vi "Anritsu1c_MT8852B_YYLL_Test.vi"(11 "YTESTER测试数据":T1={"Socket(From1)"=1, "SN"=refnum, "StopFlagRef"=refnum, "YT System Queue"=refnum}) -> (3 "YTESTER结论":T2)   [LabVIEW 2017]
doc: "VIDescription=线损设置"
uses:
  YtCommon.lvlibp/yt`Step StepBaseInput.ctl
  YtCommon.lvlibp/yt`Step StepResult.ctl
  YtCommon.lvlibp/yt`Step TestData.ctl
  YtCommon.lvlibp/yt`Step System Queue.ctl
  Step`s VIs/YYLLGeneric/variable_W.ctl
  YtCommon.lvlibp/yt`Data-Ytester Type Data.ctl
  Step`s VIs/YYLLIdea/yyllMT8852B/Anritsu_MT8852B_YYLL_Result.ctl
  <vilib>/regexp/Match Regular Expression.xnode
  YtCommon.lvlibp
panel:
  in  "YTESTER开放参数":T4={"YTESTER_BaseInput"={"isTest"=TRUE, "isSkip"=FALSE, "StepName"="AnritsuMT8852B测试", "OnPass"=enum."Next", "OnFail"=enum."Next", "ReTestNumber"=0.0}, "VISA resource name"="", "测试MAC来源"=enum."搜索测试", "指定MAC"="", "Test Timeout(s)"=30.0}
  # "#yyll 建议\n蓝牙测试繁多！测试Maybe只对生产工艺过程导致异常排筛、效率负责，无需过多专业测试。"
  # "MT8852B"
  # "Anritsu"
  # "YYLL"
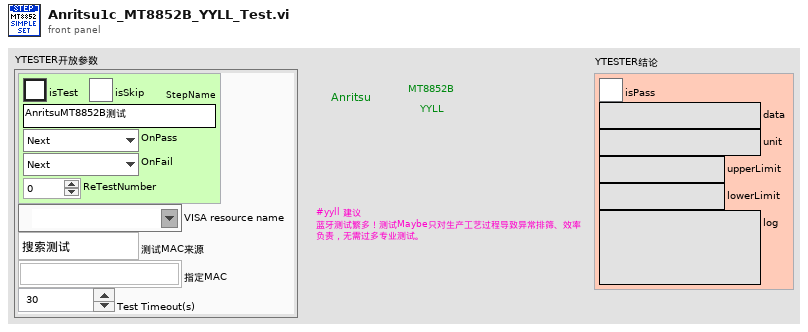
[diagram p1: front panel]
types:
  T1 = typedef "YtCommon.lvlibp/yt`Step TestData.ctl" = cluster{"Socket(From1)":i32, "SN":refnum<notifier>, "StopFlagRef":refnum<notifier>, "YT System Queue":refnum<queue>}
  T2 = typedef "YtCommon.lvlibp/yt`Step StepResult.ctl" = cluster{"isPass":bool, "data":string, "unit":string, "upperLimit":string, "lowerLimit":string, "log":string}
  T3 = typedef "YtCommon.lvlibp/yt`Step StepBaseInput.ctl" = cluster{"isTest":bool, "isSkip":bool, "StepName":string, "OnPass":enum16{"Next", "ToOVER", "Terminate"}, "OnFail":enum16{"Next", "ToOVER", "Terminate"}, "ReTestNumber":dbl}
  T4 = cluster{"YTESTER_BaseInput":T3, "VISA resource name":refnum<visa-resource-name>, "测试MAC来源":enum16{"搜索测试", "指定MAC测试"}, "指定MAC":string, "Test Timeout(s)":dbl}
  T5 = typedef "variable_W.ctl" = cluster{"YT_TYPE":T6, "TypeData":string[], "Tips":string}
  T6 = typedef "YtCommon.lvlibp/yt`Data-Ytester Type Data.ctl" = enum16{"NULL", "NUM", "BOOL", "TXT", "ENUM", "TIME", "PATH", "VISA", "COMBO", "ColorBox", "RadioBtn", "Array_NUM", "Array_BOOL", "Array_TXT", "Array_ENUM", "Array_PATH", "Array_COMBO"}
  T7 = typedef "Anritsu_MT8852B_YYLL_Result.ctl" = cluster{"AnritsuMT8852B_OP_Low_Avgpower":dbl, "AnritsuMT8852B_OP_Low_Peakpower":dbl, "AnritsuMT8852B_OP_Med_Avgpower":dbl, "AnritsuMT8852B_OP_Med_Peakpower":dbl, "AnritsuMT8852B_OP_Hig_Avgpower":dbl, "AnritsuMT8852B_OP_Hig_Peakpower":dbl, "AnritsuMT8852B_IC_Low_PositiveOffset":dbl, "AnritsuMT8852B_IC_Low_NegativeOffset":dbl, "AnritsuMT8852B_IC_Low_AvgOffset":dbl, "AnritsuMT8852B_IC_Med_PositiveOffset":dbl, "AnritsuMT8852B_IC_Med_NegativeOffset":dbl, "AnritsuMT8852B_IC_Med_AvgOffset":dbl, "AnritsuMT8852B_IC_Hig_PositiveOffset":dbl, "AnritsuMT8852B_IC_Hig_NegativeOffset":dbl, "AnritsuMT8852B_IC_Hig_AvgOffset":dbl, "AnritsuMT8852B_SS_Low_BitErrorRate":dbl, "AnritsuMT8852B_SS_Low_FrameErrorRate":dbl, "AnritsuMT8852B_SS_Med_BitErrorRate":dbl, "AnritsuMT8852B_SS_Med_FrameErrorRate":dbl, "AnritsuMT8852B_SS_Hig_BitErrorRate":dbl, "AnritsuMT8852B_SS_Hig_FrameErrorRate":dbl, "StandardLim_OP_Avg[-6,20]":bool, "StandardLim_OP_Peak[<23]":bool, "StandardLim_IC_Offset[75KHz]":bool, "StandardLim_SS_BitErrorRate[<0.1]":bool, "StandardLim_SS_FrameErrorRate[<100]":bool}
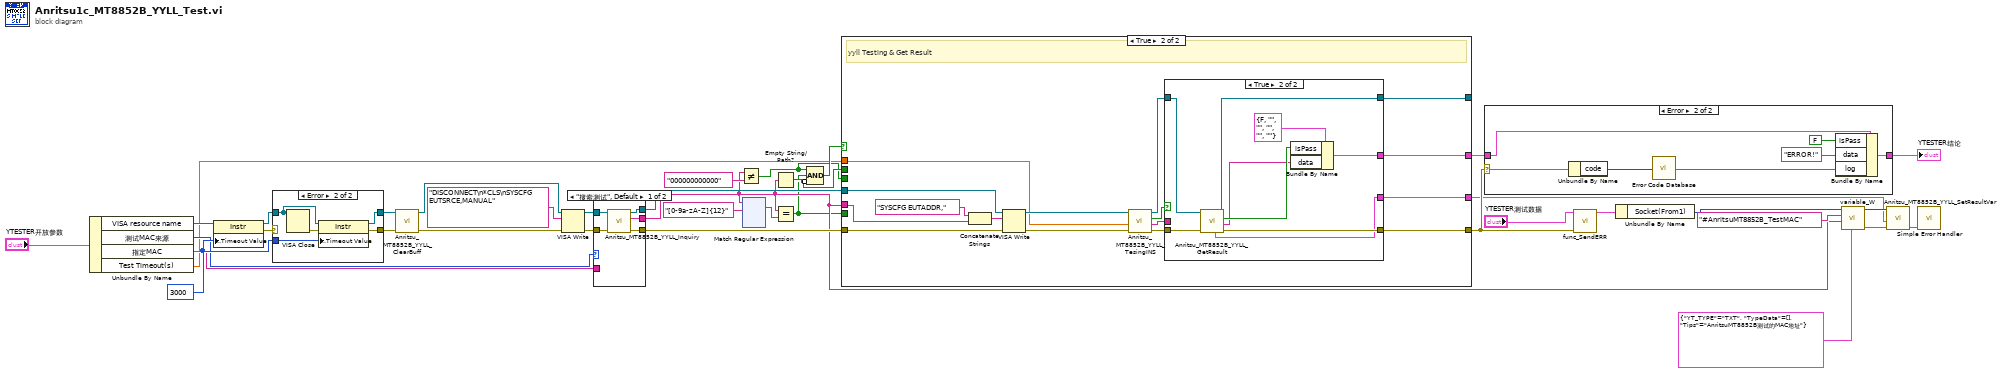
[diagram p0: block diagram]
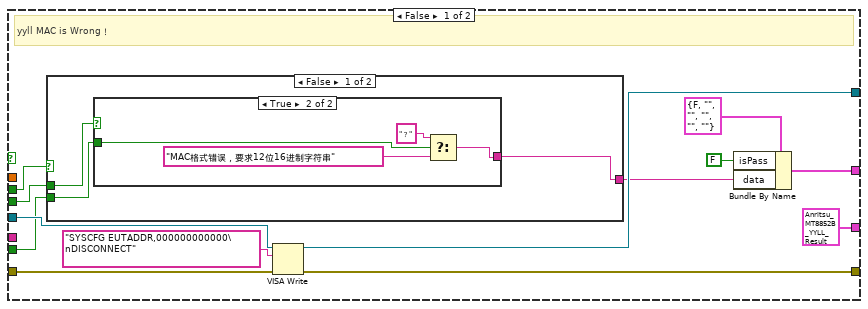
[diagram p3: hidden frame]
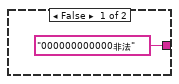
[diagram p4: hidden frame]
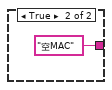
[diagram p5: hidden frame]
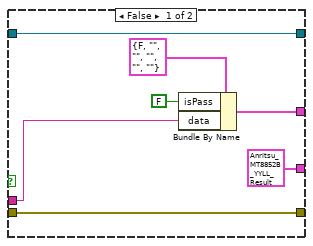
[diagram p6: hidden frame]
diagram:
  w33 = u32 3000 ("General Settings:Timeout Value")
  n1 = Unbundle By Name("YTESTER开放参数") -> ("VISA resource name"=w36:refnum<visa-resource-name>, "测试MAC来源"=w32:enum16{"搜索测试", "指定MAC测试"}, "指定MAC"=w31:string, "Test Timeout(s)"=w6:dbl)
  n2 = property class="Instr"(reference=w36, "General Settings:Timeout Value"=w33) -> (reference out=w34:refnum<visa-resource-name>, error out=w35:errorcluster)  [unwired: 1 in]
  n3 = case shown="Error" w35 {
    selector: w35 -> [w38 _]
    tunnel: w34 -> [w39 w44]
    tunnel: w33 -> [_ w42]
    tunnel: [w38 w41] -> w23
    tunnel: [w39 w40] -> w24
    frame No Error {
    }
    frame Error {
      n4 = VISA Close(VISA resource name=w44) -> (error out=w43:errorcluster)  [unwired: 1 in]
      n5 = property class="Instr"(reference=w44, error in=w43, "General Settings:Timeout Value"=w42) -> (reference out=w40:refnum<visa-resource-name>, error out=w41:errorcluster)
    }
  }
  n6 = call "Anritsu_MT8852B_YYLL_ClearBuff.vi"("error IO"=w23, "VISA resource name"=w24) -> ("error IO 2"=w21:errorcluster, "VISA resource name 2"=w19:refnum<visa-resource-name>)  [unwired: 7 in, 1 out]
  n7 = VISA Write(VISA resource name=w19, write buffer="DISCONNECT\n*CLS\nSYSCFG EUTSRCE,MANUAL", error in (no error)=w21) -> (VISA resource name out=w20:refnum<visa-resource-name>, error out=w22:errorcluster)  [unwired: 1 out]
  n8 = case shown="\"搜索测试\", Default" w32 {
    tunnel: w20 -> [w49 w51]
    tunnel: w22 -> [w48 w50]
    tunnel: [w47 w52] -> w11
    tunnel: [w46 w51] -> w27
    tunnel: [w45 w50] -> w26
    tunnel: w31 -> [_ w52]
    frame "搜索测试", Default {
      n9 = call "Anritsu_MT8852B_YYLL_Inquiry.vi"("error in (no error)"=w48, "VISA resource in"=w49) -> ("error out"=w45:errorcluster, "MAC"=w47:string, "VISA resource out"=w46:refnum<visa-resource-name>)  [unwired: 7 in]
    }
    frame "指定MAC测试" {
    }
  }
  n10 = Not Equal?(x=w11, y="000000000000") -> (x != y?=w4:bool)
  n11 = xnode "Match Regular Expression"("input string"=w11, "regular expression"="[0-9a-zA-Z]{12}") -> ("whole match"=w28:string)  [unwired: 4 in, 4 out]
  n12 = Empty String/Path?(string/path=w11) -> (empty?=w5:bool)
  n13 = Equal?(x=w11, y=w28) -> (x = y?=w3:bool)
  n14 = Compound Arithmetic op=AND(w4, w3, invert w5) -> (w30:bool)
  n15 = case shown="True" w30 {
    tunnel: w27 -> [w64 w90]
    tunnel: w26 -> [w62 w89]
    tunnel: [w63 w82] -> _
    tunnel: w11 -> [_ w88]
    tunnel: [w61 w80] -> w16
    tunnel: [T7 {"AnritsuMT8852B_OP_Low_Avgpower"=-9999.0, "AnritsuMT8852B_OP_Low_Peakpower"=-9999.0, "AnritsuMT8852B_OP_Med_Avgpower"=-9999.0, "AnritsuMT8852B_OP_Med_Peakpower"=-9999.0, "AnritsuMT8852B_OP_Hig_Avgpower"=-9999.0, "AnritsuMT8852B_OP_Hig_Peakpower"=-9999.0, "AnritsuMT8852B_IC_Low_PositiveOffset"=-9999.0, "AnritsuMT8852B_IC_Low_NegativeOffset"=-9999.0, "AnritsuMT8852B_IC_Low_AvgOffset"=-9999.0, "AnritsuMT8852B_IC_Med_PositiveOffset"=-9999.0, "AnritsuMT8852B_IC_Med_NegativeOffset"=-9999.0, "AnritsuMT8852B_IC_Med_AvgOffset"=-9999.0, "AnritsuMT8852B_IC_Hig_PositiveOffset"=-9999.0, "AnritsuMT8852B_IC_Hig_NegativeOffset"=-9999.0, "AnritsuMT8852B_IC_Hig_AvgOffset"=-9999.0, "AnritsuMT8852B_SS_Low_BitErrorRate"=-9999.0, "AnritsuMT8852B_SS_Low_FrameErrorRate"=-9999.0, "AnritsuMT8852B_SS_Med_BitErrorRate"=-9999.0, "AnritsuMT8852B_SS_Med_FrameErrorRate"=-9999.0, "AnritsuMT8852B_SS_Hig_BitErrorRate"=-9999.0, "AnritsuMT8852B_SS_Hig_FrameErrorRate"=-9999.0, "StandardLim_OP_Avg[-6,20]"=FALSE, "StandardLim_OP_Peak[<23]"=FALSE, "StandardLim_IC_Offset[75KHz]"=FALSE, "StandardLim_SS_BitErrorRate[<0.1]"=FALSE, "StandardLim_SS_FrameErrorRate[<100]"=FALSE} ("Anritsu_MT8852B_YYLL_Result") w78] -> w8
    tunnel: [w57 w77] -> w7
    tunnel: w6 -> [_ w75]
    tunnel: w5 -> [w56 _]
    tunnel: w4 -> [w54 _]
    tunnel: w3 -> [w53 _]
    frame False {
      # "yyll MAC is Wrong！"
      n16 = case shown="False" w56 {
        tunnel: [w67 "空MAC" ("data")] -> w55
        tunnel: w54 -> [w68 _]
        tunnel: w53 -> [w66 _]
        frame False {
          n17 = case shown="True" w68 {
            tunnel: ["000000000000非法" ("y") w71] -> w67
            tunnel: w66 -> [_ w73]
            frame False {
            }
            frame True {
              n18 = Select(t="？" ("y"), s=w73, f="MAC格式错误，要求12位16进制字符串" ("y")) -> (s? t:f=w71:string)
            }
          }
        }
        frame True {
        }
      }
      n19 = VISA Write(VISA resource name=w64, write buffer="SYSCFG EUTADDR,000000000000\nDISCONNECT" ("Format String"), error in (no error)=w62) -> (VISA resource name out=w63:refnum<visa-resource-name>, error out=w61:errorcluster)  [unwired: 1 out]
      n20 = Bundle By Name(cluster=T2 {"isPass"=FALSE, "data"="", "unit"="", "upperLimit"="", "lowerLimit"="", "log"=""} ("Result"), "isPass"=FALSE, "data"=w55) -> (w57:T2)
    }
    frame True {
      # "yyll Testing & Get Result"
      n21 = Concatenate Strings("SYSCFG EUTADDR," ("Format String"), w88) -> (w86:string)
      n22 = VISA Write(VISA resource name=w90, write buffer=w86, error in (no error)=w89) -> (VISA resource name out=w85:refnum<visa-resource-name>, error out=w84:errorcluster)  [unwired: 1 out]
      n23 = call "Anritsu_MT8852B_YYLL_TesingINS.vi"("error in"=w84, "Test Timeout"=w75, "VISA resource in"=w85) -> ("error out"=w81:errorcluster, "TestStopString"=w76:string, "test done to read"=w79:bool, "VISA resource out"=w83:refnum<visa-resource-name>)  [unwired: 5 in]
      n24 = case shown="True" w79 {
        tunnel: w83 -> [w96 w106]
        tunnel: [w96 w105] -> w82
        tunnel: w81 -> [w95 w104]
        tunnel: [w95 w103] -> w80
        tunnel: [T7 {"AnritsuMT8852B_OP_Low_Avgpower"=-9999.0, "AnritsuMT8852B_OP_Low_Peakpower"=-9999.0, "AnritsuMT8852B_OP_Med_Avgpower"=-9999.0, "AnritsuMT8852B_OP_Med_Peakpower"=-9999.0, "AnritsuMT8852B_OP_Hig_Avgpower"=-9999.0, "AnritsuMT8852B_OP_Hig_Peakpower"=-9999.0, "AnritsuMT8852B_IC_Low_PositiveOffset"=-9999.0, "AnritsuMT8852B_IC_Low_NegativeOffset"=-9999.0, "AnritsuMT8852B_IC_Low_AvgOffset"=-9999.0, "AnritsuMT8852B_IC_Med_PositiveOffset"=-9999.0, "AnritsuMT8852B_IC_Med_NegativeOffset"=-9999.0, "AnritsuMT8852B_IC_Med_AvgOffset"=-9999.0, "AnritsuMT8852B_IC_Hig_PositiveOffset"=-9999.0, "AnritsuMT8852B_IC_Hig_NegativeOffset"=-9999.0, "AnritsuMT8852B_IC_Hig_AvgOffset"=-9999.0, "AnritsuMT8852B_SS_Low_BitErrorRate"=-9999.0, "AnritsuMT8852B_SS_Low_FrameErrorRate"=-9999.0, "AnritsuMT8852B_SS_Med_BitErrorRate"=-9999.0, "AnritsuMT8852B_SS_Med_FrameErrorRate"=-9999.0, "AnritsuMT8852B_SS_Hig_BitErrorRate"=-9999.0, "AnritsuMT8852B_SS_Hig_FrameErrorRate"=-9999.0, "StandardLim_OP_Avg[-6,20]"=FALSE, "StandardLim_OP_Peak[<23]"=FALSE, "StandardLim_IC_Offset[75KHz]"=FALSE, "StandardLim_SS_BitErrorRate[<0.1]"=FALSE, "StandardLim_SS_FrameErrorRate[<100]"=FALSE} ("Anritsu_MT8852B_YYLL_Result") w102] -> w78
        tunnel: [w92 w100] -> w77
        tunnel: w76 -> [w91 _]
        frame False {
          n25 = Bundle By Name(cluster=T2 {"isPass"=FALSE, "data"="", "unit"="", "upperLimit"="", "lowerLimit"="", "log"=""} ("Result"), "isPass"=FALSE, "data"=w91) -> (w92:T2)
        }
        frame True {
          n26 = call "Anritsu_MT8852B_YYLL_GetResult.vi"("error in"=w104, "VISA resource in"=w106) -> ("error out"=w103:errorcluster, "ValidString"=w98:string, "Valid OK?"=w99:bool, "VISA resource out"=w105:refnum<visa-resource-name>, "Anritsu_MT8852B_YYLL_Result"=w102:T7)  [unwired: 5 in]
          n27 = Bundle By Name(cluster=T2 {"isPass"=FALSE, "data"="", "unit"="", "upperLimit"="", "lowerLimit"="", "log"=""} ("Result"), "isPass"=w99, "data"=w98) -> (w100:T2)
        }
      }
    }
  }
  n28 = case shown="Error" w16 {
    selector: w16 -> [_ w114]
    tunnel: w7 -> [w107 w112]
    tunnel: [w107 w110] -> w15
    frame No Error {
    }
    frame Error {
      n29 = Unbundle By Name(w114) -> ("code"=w113:i32)
      n30 = call <vilib>:"Error Code Database.vi"("Error Code"=w113) -> ("Error Text"=w111:string)
      n31 = Bundle By Name(cluster=w112, "isPass"=FALSE, "data"="ERROR!", "log"=w111) -> (w110:T2)
    }
  }
  "YTESTER结论" <- w15
  n32 = call "func_SendERR.vi"("ERR (String\\Errclust)"=w16, "YTESTER测试数据 in"="YTESTER测试数据") -> ("YTESTER测试数据 out"=w14:T1)  [unwired: 9 in]
  n33 = Unbundle By Name(w14) -> ("Socket(From1)"=w13:i32)
  n34 = call "variable_W.vi"("附加的Information"=T5 {"YT_TYPE"=enum."TXT", "TypeData"=[], "Tips"="AnritsuMT8852B测试的MAC地址"}, "待写入池的输入控件"=w11, "待写入池变量名称"="#AnritsuMT8852B_TestMAC", "函数池名称 in"=w13) -> ("error out"=w2:errorcluster, "函数池名称 out"=w9:i32)  [unwired: 5 in, 1 out]
  n35 = call "Anritsu_MT8852B_YYLL_SetResultVar.vi"("error in (no error)"=w2, "Anritsu_MT8852B_YYLL_Result"=w8, "函数池名称"=w9) -> ("error out"=w1:errorcluster)  [unwired: 8 in]
  n36 = call <vilib>:"Simple Error Handler.vi"("error in (no error)"=w1) -> ()  [unwired: 4 in, 5 out]
